vi "Fit Model to Plot Core.vi"(0 "Fit Plot Information":T11={"XY Graph Ref"=refnum, "Mouse Coordinates"={"X"=0.0, "Y"=0.0}, "Fit Model"=enum."Select a Fit Model...", "Plot Index"=-1}, 2 "Display Plots (T)":bool=TRUE, 5 "Fit Settings":T6={"Use Original Plot # Points"=FALSE, "# Fit Plot Points"=0, "Fitting Method"=enum."Least Square", "Weighted Fit"=enum."Unweighted", "Show All Fit Components"=FALSE, "Axis Type"=0, "Show Fit Residuals"=TRUE, "Residual Type"=enum."Standard", "Fitting Algorithm"=enum."Levenberg-Marquardt", "Show Confidence Interval"=FALSE, "Confidence Level"=95.0} {"Confidence Level" min=0.0 max=100.0; "Axis Type" items=["Linear", "Logarithmic"]}, 7 "Termination Criteria":T5={"Max Iterations"=1000, "Max Function Calls"=10000, "Max Time"=1000.0, "Function Tolerance"=1e-06, "Parameter Tolerance"=1e-06, "Gradient Tolerance"=1e-06, "Min Lambda"=1e-06, "Max Lambda"=1000000.0, "Initial Tick Count"=0}, 9 "Fit Model Information":T2, 11 "error in (no error)":errorcluster, 12 "Send Graph to Notebook?":bool) -> (3 "Plot Name":string, 4 "Array of Plots (Fit, Components, Residuals)":cluster{"X Array":dbl[], "Y Array":dbl[]}[](array[cluster]), 6 "best nonlinear fit":dbl[](array[numeric]), 8 "Fit Output Data":T1, 14 "Fitting Algorithm":T4, 15 "error out":errorcluster)   [LabVIEW 2021, in "Fits.lvlib"]
uses:
  Fits.lvlib
  Fit Plot Request Information.ctl
  <vilib>/Utility/miscctls.llb/LVPointDoubleTypeDef.ctl
  Fit Models.ctl
  Fit Settings.ctl
  Nonlinear Fit Method.ctl
  Ramp Type.ctl
  Residual Type.ctl
  Non-linear Fitting Algorithm.ctl
  My Fit Stopping Criteria.ctl
  Fit Model Information.ctl
  Fit Output Data.ctl
  Graphs/Single Plot Style 2.ctl
  Notebook/Notebook.lvlib
  Graphs/XY Graph/XY Graph Add-Ons.lvlib
  Graphs/Graphs.lvlib
  IRF(X)PSED/Fit Weights Type v2.ctl
panel:
  out "Fitted Plot":cluster{"X Array":dbl[], "Y Array":dbl[]}
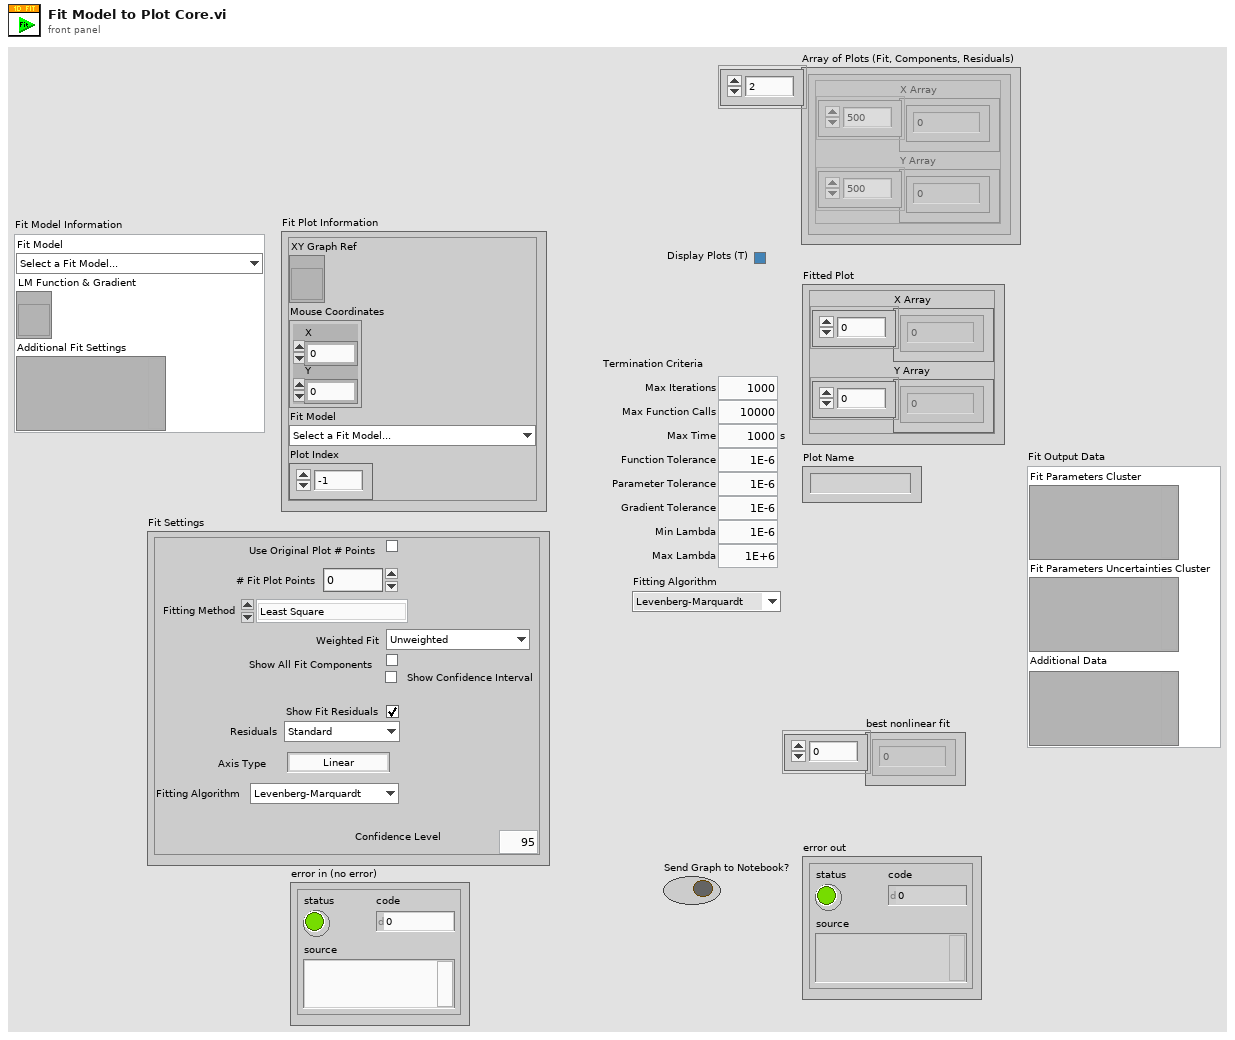
[diagram p1: front panel]
types:
  T1 = typedef "Fits.lvlib/Fit Output Data.ctl" = cluster{"Fit Parameters Cluster":variant, "Fit Parameters Uncertainties Cluster":variant, "Additional Data":variant}
  T2 = typedef "Fits.lvlib/Fit Model Information.ctl" = cluster{"Fit Model":T3, "LM Function & Gradient":refnum<vi>, "Additional Fit Settings":variant}
  T3 = typedef "Fits.lvlib/Fit Models.ctl" = enum16{"Select a Fit Model...", "           Single Peak", "Gaussian", "Asymmetric Gaussian", "Lorentzian", "Asymmetric Lorentzian", "Gaussian/Lorentzian", "Lorentzian/Gaussian", "           Double Peak", "Two Gaussians", "Two Asymmetric Gaussians", "Two H-Connected Gaussians", "Two T-Connected Gaussians", "Two H-Connected Asymmetric Gaussians", "Two T-Connected Asymmetric Gaussians", "           Triple Peak", "Three Gaussians", "Three Asymmetric Gaussians", "              Decays", "1-Exponential", "IRF*PSED", "2-Exponentials", "            Power Law", "Power Law", "Power Law with Offset", "               ACF", "2D Gaussian ACF", "2D Gaussian + Blinking ACF", "2D Gaussian + Flow ACF", "3D Gaussian ACF", "3D Gaussian + Blinking ACF", "             Multiplot", "2D Gaussian ACF & 2D Gaussian + Flow ACF"}
  T4 = typedef "Fits.lvlib/Non-linear Fitting Algorithm.ctl" = enum16{"Levenberg-Marquardt", "Trust-Region Dogleg"}
  T5 = typedef "Fits.lvlib/My Fit Stopping Criteria.ctl" = cluster{"Max Iterations":i32, "Max Function Calls":i32, "Max Time":dbl[unit], "Function Tolerance":dbl, "Parameter Tolerance":dbl, "Gradient Tolerance":dbl, "Min Lambda":dbl, "Max Lambda":dbl, "Initial Tick Count":u32}
  T6 = typedef "Fits.lvlib/Fit Settings.ctl" = cluster{"Use Original Plot # Points":bool, "# Fit Plot Points":u32, "Fitting Method":T7, "Weighted Fit":T8, "Show All Fit Components":bool, "Axis Type":T9, "Show Fit Residuals":bool, "Residual Type":T10, "Fitting Algorithm":T4, "Show Confidence Interval":bool, "Confidence Level":dbl}
  T7 = typedef "Fits.lvlib/Nonlinear Fit Method.ctl" = enum16{"Least Square", "Least Absolute Residual", "Bisquare", "MLE"}
  T8 = typedef "Fits.lvlib/Fit Weights Type v2.ctl" = enum16{"Unweighted", "1/Variance (Neyman)", "1/Variance (Pearson)", "Best of All"}
  T9 = typedef "Fits.lvlib/Ramp Type.ctl" = u16
  T10 = typedef "Fits.lvlib/Residual Type.ctl" = enum16{"Standard", "Normalized", "Reduced"}
  T11 = typedef "Fits.lvlib/Fit Plot Request Information.ctl" = cluster{"XY Graph Ref":refnum<vi>, "Mouse Coordinates":T12, "Fit Model":T3, "Plot Index":i32}
  T12 = typedef "LVPointDoubleTypeDef.ctl" = cluster{"X":dbl, "Y":dbl}
  T13 = typedef "Graphs.lvlib/Single Plot Style 2.ctl" = cluster{"Plot Style":enum16{"unchanged", "Line", "Symbol", "Line + Symbol", "Histogram", "Histogram + Symbol"}, "Histogram Type":enum16{"unchanged", "Left Bound", "Center", "Right Bound"}, "Line Tickness":enum16{"unchanged", "Thin", "1 pixel", "2 pixel", "3 pixel", "4 pixel", "5 pixel"}, "Line Style":enum16{"unchanged", "Plain", "Long Dash", "Short Dash", "Long-Short Dash", "Long-Short-Short Dash"}, "Point Style":enum16{"unchanged", "None", "Empty Circle", "Filled Circle", "Thick Circle", "Dotted Circle", "Empty Square", "Filled Square", "Thick Square", "Dotted Square", "Small Filled Square", "Dot", "Cross", "Tiny Cross", "Large X", "Small x", "Diamond", "Small Empty Square"}, "Line Color":u32, "Line Color defined?":bool, "Point Color":u32, "Point Color defined?":bool, "Anti-aliased":bool}
  T14 = typedef "XY Graph Add-Ons.lvlib/XY Graph Plot Data.ctl" = cluster{"X Array":dbl[], "Y Array":dbl[]}
  T15 = typedef "Fits.lvlib/Fit Output Arrays.ctl" = cluster{"Clipped Plot X Array":dbl[], "Clipped Plot Y Array":dbl[], "Weight Array":dbl[], "Best Nonlinear Fit":dbl[], "Best Fit Parameters":dbl[]}
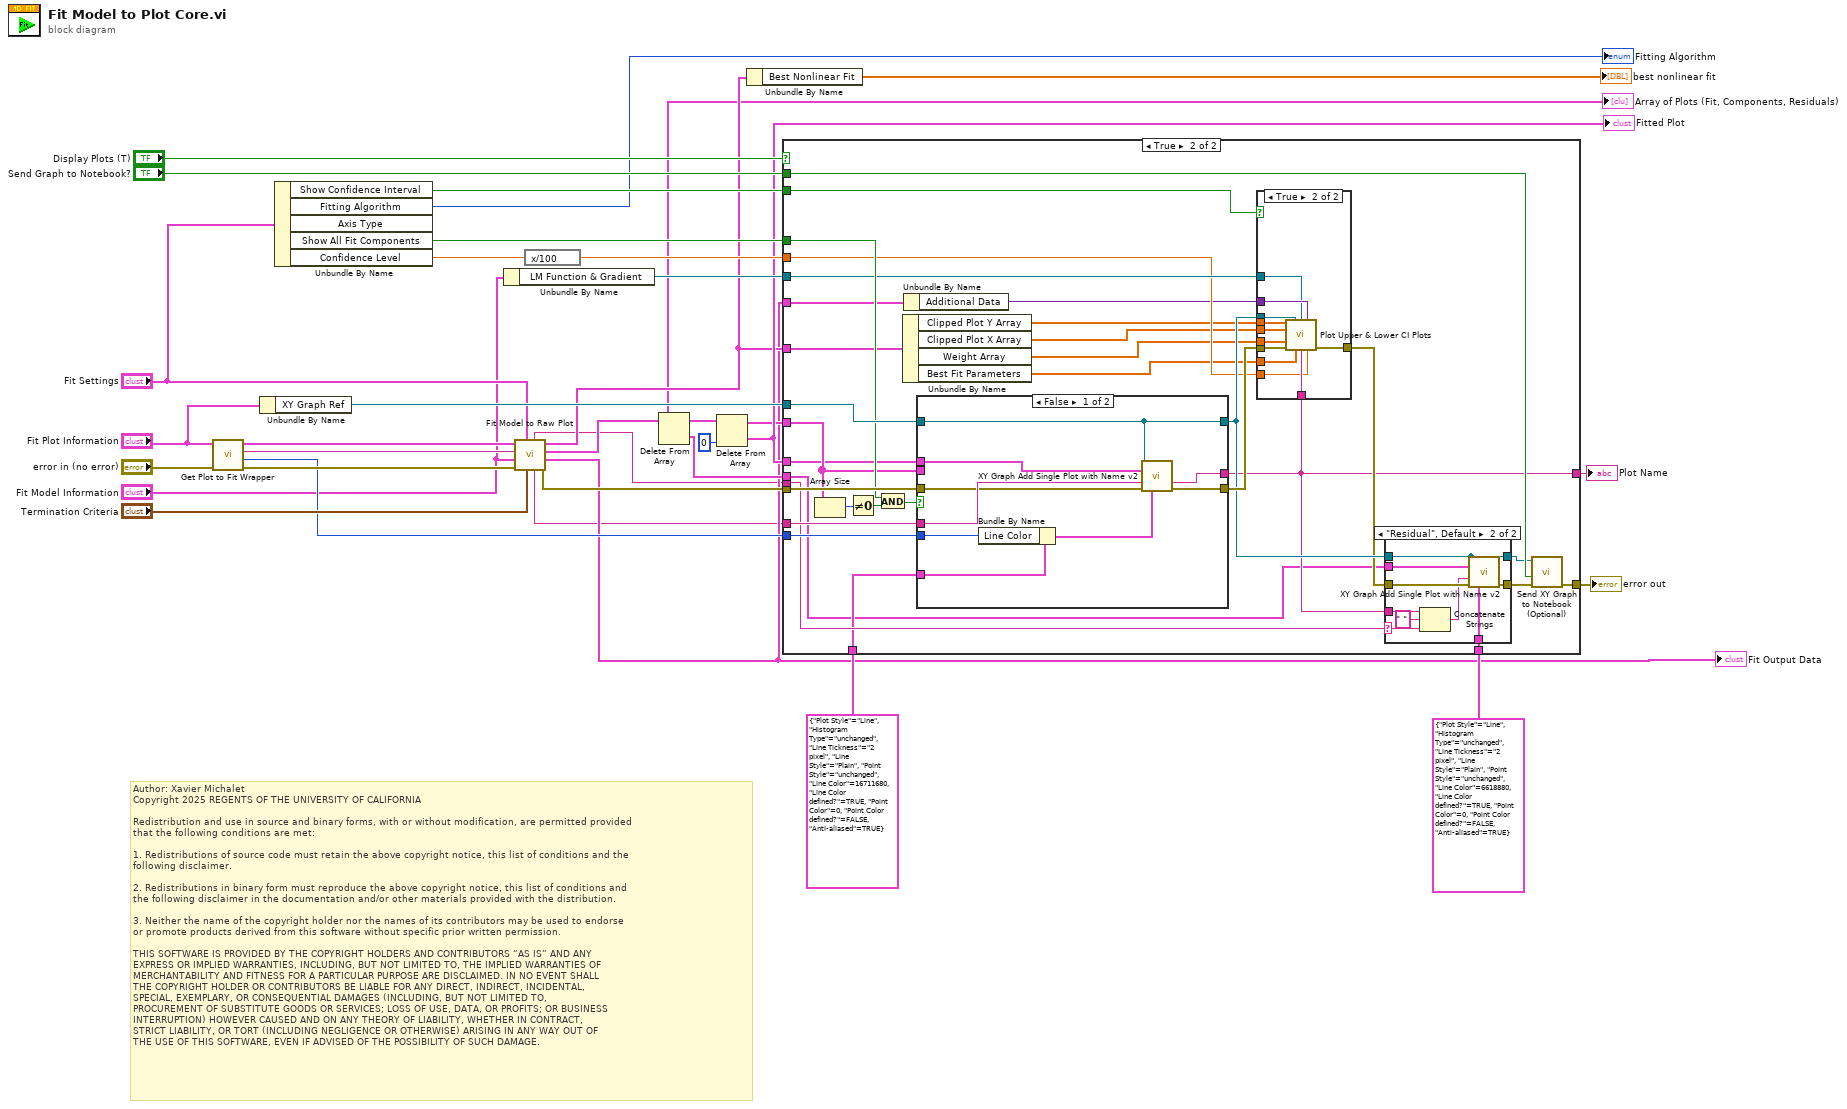
[diagram p0: block diagram]
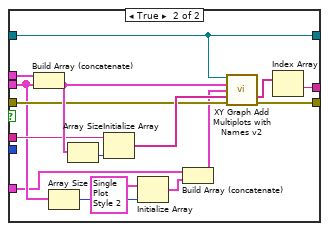
[diagram p5: hidden frame]
diagram:
  # "Author: Xavier Michalet\nCopyright 2025 REGENTS OF THE UNIVERSITY OF CALIFORNIA\n\nRedistribution and use in source and binary forms, with or without modification, are permitted provided\nthat the following conditions are met:\n\n1. Redistributions of source code must retain the above copyright notice, this list of conditions and the\nfollowing disclaimer.\n\n2. Redistributions in binary form must reproduce the above copyright notice, this list of conditions and\nthe following disclaimer in the documentation and/or other materials provided with the distribution.\n\n3. Neither the name of the copyright holder nor the names of its contributors may be used to endorse \nor promote products derived from this software without specific prior written permission.\n\nTHIS SOFTWARE IS PROVIDED BY THE COPYRIGHT HOLDERS AND CONTRIBUTORS “AS IS” AND ANY \nEXPRESS OR IMPLIED WARRANTIES, INCLUDING, BUT NOT LIMITED TO, THE IMPLIED WARRANTIES OF\nMERCHANTABILITY AND FITNESS FOR A PARTICULAR PURPOSE ARE DISCLAIMED. IN NO EVENT SHALL\nTHE COPYRIGHT HOLDER OR CONTRIBUTORS BE LIABLE FOR ANY DIRECT, INDIRECT, INCIDENTAL, \nSPECIAL, EXEMPLARY, OR CONSEQUENTIAL DAMAGES (INCLUDING, BUT NOT LIMITED TO, \nPROCUREMENT OF SUBSTITUTE GOODS OR SERVICES; LOSS OF USE, DATA, OR PROFITS; OR BUSINESS\nINTERRUPTION) HOWEVER CAUSED AND ON ANY THEORY OF LIABILITY, WHETHER IN CONTRACT, \nSTRICT LIABILITY, OR TORT (INCLUDING NEGLIGENCE OR OTHERWISE) ARISING IN ANY WAY OUT OF\nTHE USE OF THIS SOFTWARE, EVEN IF ADVISED OF THE POSSIBILITY OF SUCH DAMAGE."
  n1 = call "Get Plot to Fit Wrapper.vi"("error in (no error)"="error in (no error)", "Fit Plot Information"="Fit Plot Information") -> ("error out"=w22:errorcluster, "Plot Color"=w16:u32, "Plot Name"=w24:string, "Clipped Plot"=w23:T14)  [unwired: 3 in, 3 out]
  n2 = Unbundle By Name("Fit Plot Information") -> ("XY Graph Ref"=w25:refnum<vi>)
  n3 = Unbundle By Name("Fit Settings") -> ("Show Confidence Interval"=w20:bool, "Fitting Algorithm"=→"Fitting Algorithm":T4, "Show All Fit Components"=w33:bool, "Confidence Level"=w18:dbl)  [unwired: 1 out]
  n4 = Unbundle By Name("Fit Model Information") -> ("LM Function & Gradient"=w12:refnum<vi>)
  n5 = call "Fit Model to Raw Plot.vi"("Termination Criteria"="Termination Criteria", "Fit Settings"="Fit Settings", "error in (no error)"=w22, "Fit Model Information"="Fit Model Information", "Plot Name (Plot)"=w24, "Plot"=w23) -> ("error out"=w34:errorcluster, "Fit Output Data"=w3:T1, "Array of Plots (Fit, n Components, Residuals)"=w4:cluster{"X Array":dbl[], "Y Array":dbl[]}[], "Fit Output Arrays"=w5:T15, "Fit Plot Name"=w1:string, "Residual Type"=w2:string)
  "Array of Plots (Fit, Components, Residuals)" <- w4
  "Fit Output Data" <- w3
  n6 = expression code="x/100"(w18) -> (w14:dbl)
  n7 = Delete From Array(array=w4) -> (deleted portion=w11:cluster{"X Array":dbl[], "Y Array":dbl[]}, array with subset deleted=w10:cluster{"X Array":dbl[], "Y Array":dbl[]}[])  [unwired: 2 in]
  n8 = Delete From Array(array=w10, index=0) -> (deleted portion=w8:cluster{"X Array":dbl[], "Y Array":dbl[]}, array with subset deleted=w7:cluster{"X Array":dbl[], "Y Array":dbl[]}[])  [unwired: 1 in]
  "Fitted Plot" <- w8
  n9 = Unbundle By Name(w5) -> ("Best Nonlinear Fit"=→"best nonlinear fit":dbl[])
  n10 = case shown="True" "Display Plots (T)" {
    tunnel: w1 -> [w35 w68]
    tunnel: w16 -> [_ w67]
    tunnel: w34 -> [w36 w66]
    tunnel: w25 -> [_ w65]
    tunnel: w33 -> [_ w62]
    tunnel: w8 -> [_ w51]
    tunnel: w7 -> [_ w60]
    tunnel: "Send Graph to Notebook?" -> [_ w59]
    tunnel: [w36 w58] -> w30
    tunnel: w2 -> [_ w50]
    tunnel: w11 -> [_ w45]
    tunnel: [w35 w49] -> w29
    tunnel: w12 -> [_ w52]
    tunnel: T13 {"Plot Style"=enum."Line", "Histogram Type"=enum."unchanged", "Line Tickness"=enum."2 pixel", "Line Style"=enum."Plain", "Point Style"=enum."unchanged", "Line Color"=16711680, "Line Color defined?"=TRUE, "Point Color"=0, "Point Color defined?"=FALSE, "Anti-aliased"=TRUE} ("Plot Style") -> [_ w48]
    tunnel: w20 -> [_ w47]
    tunnel: T13 {"Plot Style"=enum."Line", "Histogram Type"=enum."unchanged", "Line Tickness"=enum."2 pixel", "Line Style"=enum."Plain", "Point Style"=enum."unchanged", "Line Color"=6618880, "Line Color defined?"=TRUE, "Point Color"=0, "Point Color defined?"=FALSE, "Anti-aliased"=TRUE} ("Plot Style") -> [_ w46]
    tunnel: w14 -> [_ w44]
    tunnel: w3 -> [_ w43]
    tunnel: w5 -> [_ w41]
    frame False {
    }
    frame True {
      n11 = Array Size(array=w60) -> (size(s)=w64:i32)
      n12 = Not Equal To 0?(x=w64) -> (x != 0?=w63:bool)
      n13 = And(x=w62, y=w63) -> (x .and. y?=w61:bool)
      n14 = Unbundle By Name(w41) -> ("Clipped Plot Y Array"=w40:dbl[], "Clipped Plot X Array"=w39:dbl[], "Weight Array"=w38:dbl[], "Best Fit Parameters"=w37:dbl[])
      n15 = Unbundle By Name(w43) -> ("Additional Data"=w42:variant)
      n16 = case shown="False" w61 {
        tunnel: w68 -> [w100 w108]
        tunnel: [w99 w110] -> w55
        tunnel: [w98 w109] -> w49
        tunnel: w67 -> [w93 _]
        tunnel: w66 -> [w97 w111]
        tunnel: w65 -> [w95 w107]
        tunnel: w51 -> [w96 w112]
        tunnel: w60 -> [_ w106]
        tunnel: [w95 w107] -> w54
        tunnel: w48 -> [w92 w103]
        frame False {
          n17 = Bundle By Name(cluster=w92, "Line Color"=w93) -> (w94:T13)
          n18 = call "XY Graph Add Single Plot with Name v2.vi"("XYGraph Ref in"=w95, "Plot"=w96, "Plot Name (\"Plot\")"=w100, "error in (no error)"=w97, "Plot Style"=w94) -> ("Plot Name"=w98:string, "error out"=w99:errorcluster)  [unwired: 7 in, 2 out]
        }
        frame True {
          n19 = Build Array (concatenate)(w112, w106) -> (w116:cluster{"X Array":dbl[], "Y Array":dbl[]}[])
          n20 = Array Size(array=w106) -> (size(s)=w105:i32)
          n21 = Array Size(array=w116) -> (size(s)=w115:i32)
          n22 = Initialize Array(w108, w115) -> (w114:string[])
          n23 = Initialize Array(T13 {"Plot Style"=enum."unchanged", "Histogram Type"=enum."Left Bound", "Line Tickness"=enum."unchanged", "Line Style"=enum."unchanged", "Point Style"=enum."unchanged", "Line Color"=0, "Line Color defined?"=FALSE, "Point Color"=0, "Point Color defined?"=FALSE, "Anti-aliased"=FALSE} ("Plot Style"), w105) -> (w102:T13[])
          n24 = Build Array (concatenate)(w103, w102) -> (w101:T13[])
          n25 = call "XY Graph Add Multiplots with Names v2.vi"("XYGraph in"=w107, "Array of Plots"=w116, "Plots Metadata"=w101, "Array of Plot Names (\"Plot\")"=w114, "error in (no error)"=w111) -> ("Added Plot Names"=w113:string[], "error out"=w110:errorcluster)  [unwired: 6 in, 3 out]
          n26 = Index Array(array=w113) -> (element=w109:string)  [unwired: 1 in]
        }
      }
      n27 = case shown="True" w47 {
        tunnel: w55 -> [w69 w80]
        tunnel: w54 -> [_ w79]
        tunnel: [w69 w78] -> w53
        tunnel: w42 -> [_ w77]
        tunnel: w52 -> [_ w76]
        tunnel: w40 -> [_ w75]
        tunnel: w39 -> [_ w74]
        tunnel: w38 -> [_ w71]
        tunnel: w37 -> [_ w72]
        tunnel: w49 -> [_ w73]
        tunnel: w44 -> [_ w70]
        frame False {
        }
        frame True {
          n28 = call "Plot Upper & Lower CI Plots.vi"("Y Array"=w75, "XY Graph Ref"=w79, "VI in"=w76, "Additional LM Data"=w77, "X Array"=w74, "Weight Array"=w71, "error in (no error)"=w80, "best fit parameters"=w72, "Fitted Plot Name"=w73, "confidence level (0.68)"=w70) -> ("error out"=w78:errorcluster)  [unwired: 5 in]
        }
      }
      n29 = case shown="\"Residual\", Default" w50 {
        selector: w50 -> [_ w86]
        tunnel: w45 -> [_ w90]
        tunnel: w49 -> [_ w87]
        tunnel: w54 -> [w82 w88]
        tunnel: w53 -> [w81 w91]
        tunnel: [w81 w89] -> w57
        tunnel: [w82 w88] -> w56
        tunnel: w46 -> [_ w83]
        frame "" {
        }
        frame "Residual", Default {
          n30 = Concatenate Strings(w87, " " ("string"), w86) -> (w84:string)
          n31 = call "XY Graph Add Single Plot with Name v2.vi"("XYGraph Ref in"=w88, "Plot"=w90, "Plot Name (\"Plot\")"=w84, "error in (no error)"=w91, "Plot Style"=w83) -> ("error out"=w89:errorcluster)  [unwired: 7 in, 3 out]
        }
      }
      n32 = call "Send XY Graph to Notebook (Optional).vi"("error in (no error)"=w57, "Send Graph to Notebook?"=w59, "XYGraph in"=w56) -> ("error out"=w58:errorcluster)  [unwired: 8 in]
    }
  }
  "error out" <- w30
  "Plot Name" <- w29
